vi "calculate checkpoint duration.vi"(8 "error in (no error)":errorcluster, 11 "Autofocus in":refnum<class "Autofocus.lvclass">) -> (0 "error out":errorcluster, 3 "Autofocus out":refnum<class "Autofocus.lvclass">)   [LabVIEW 2012, in "Autofocus.lvclass"]
uses:
  Autofocus.lvclass
  Autofocus.lvclass/Autofocus.ctl
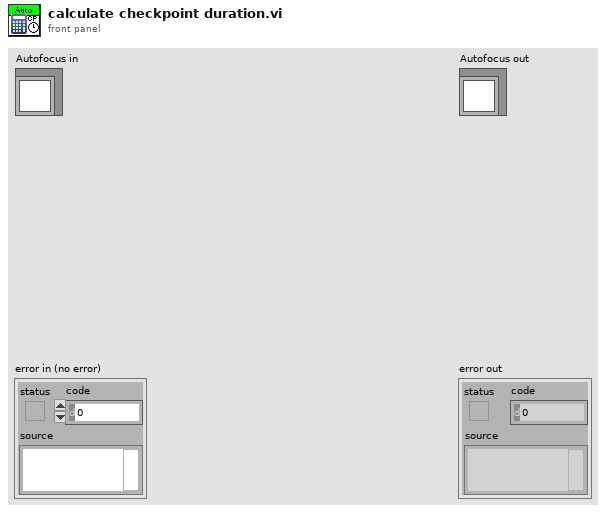
[diagram p1: front panel]
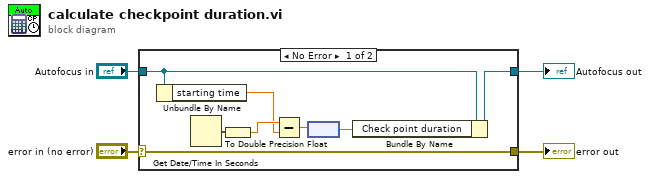
[diagram p0: block diagram]
diagram:
  n1 = case shown="No Error" "error in (no error)" {
    selector: "error in (no error)" -> [w12 w14]
    tunnel: [w12 w14] -> w3
    tunnel: [w5 w13] -> w1
    tunnel: "Autofocus in" -> [w6 w13]
    frame No Error {
      n2 = Unbundle By Name(w6) -> ("starting time"=w8:dbl)
      n3 = Get Date/Time In Seconds() -> (seconds since 1Jan1904=w11:timestamp)
      n4 = To Double Precision Float(number=w11) -> (double precision float=w9:dbl)
      n5 = Subtract(x=w9, y=w8) -> (x-y=w10:dbl)
      n6 = node(w10) -> (w7:dbl[unit])
      n7 = Bundle By Name(cluster=w6, "Check point duration"=w7) -> (w5:refnum<class "Autofocus.lvclass">)
    }
    frame Error {
    }
  }
  "error out" <- w3
  "Autofocus out" <- w1
